vi "Test Find Chessboard Corners.vi"(8 "error in (no error)":errorcluster, 11 "Test Case In":refnum<class "02_FeatureDetection.lvclass">) -> (0 "error out":errorcluster, 3 "Test Case Out":refnum<class "02_FeatureDetection.lvclass">)   [LabVIEW 2020, in "test.lvlib" / "02_FeatureDetection.lvclass"]
uses:
  02_FeatureDetection.lvclass
  02_FeatureDetection.lvclass/02_FeatureDetection.ctl
  image/image.lvlib
  ar/ar.lvlib
  <vilib>/Astemes/LUnit/Test Case.lvclass
  common/Image Size (Integer).ctl
  common/common.lvlib
  ar/Chessboard Corner Info.ctl
  ar/Find Chessboard Corners (Greyscale).vi
  image/Draw Circle (Greyscale).vi
  image/Draw Image to Picture (Greyscale).vi
  common/Image Point (Float).ctl
  image/Interpolation Mode.ctl
  image/New Image (Greyscale Preallocated).vi
  image/Resize (Greyscale).vi
  image/New Image (Greyscale Array).vi
  C:/Program Files (x86)/National Instruments/LabVIEW 2020/vi.lib/Astemes/LUnit/Test Case.lvclass
  C:/Program Files (x86)/National Instruments/LabVIEW 2020/vi.lib/Astemes/LUnit/LUnit Runnable.lvclass
  C:/serenial/lib/g-augmented-reality-toolkit/LabVIEW/test/FeatureDetection/02_FeatureDetection.lvclass
panel:
  out "Points":T1[](array[typedef])
  out "Points Refined":T1[](array[typedef])
  out "Picture":picture
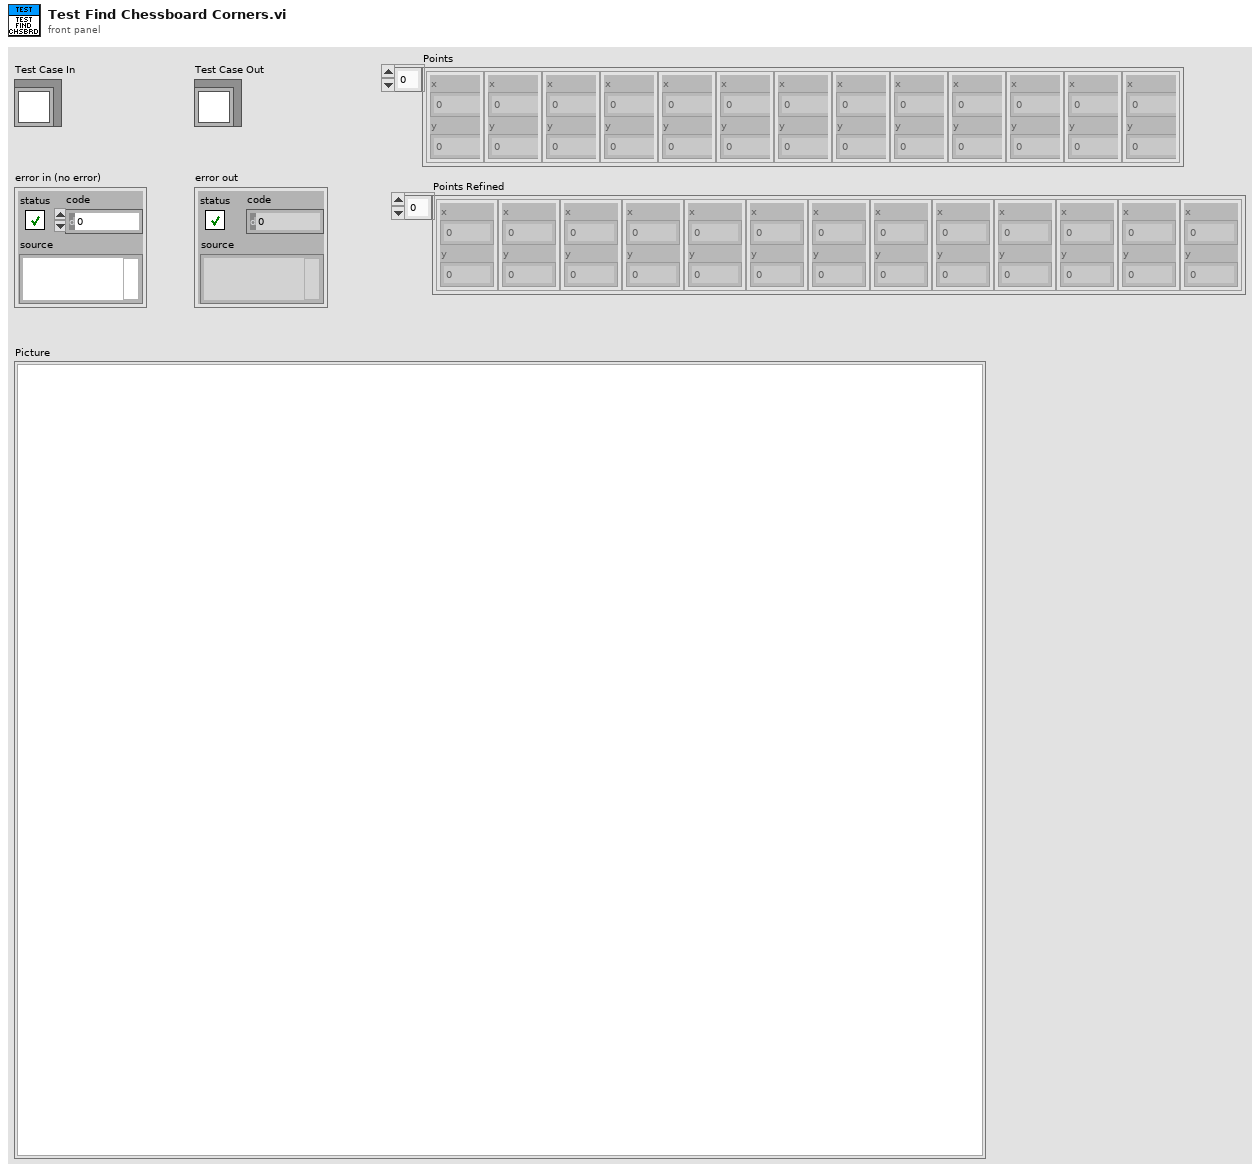
[diagram p1: front panel]
types:
  T1 = typedef "common.lvlib/Image Point (Float).ctl" = cluster{"x":dbl, "y":dbl}
  T2 = typedef "image.lvlib/Interpolation Mode.ctl" = enum8{"NEAREST", "LINEAR", "CUBIC", "AREA", "LANCZOS", "LINEAR_EXACT", "NEAREST_EXACT", "MAX"}
  T3 = typedef "ar.lvlib/Chessboard Corner Info.ctl" = cluster{"Points Per Row":u8, "Points Per Col":u8}
  T4 = typedef "common.lvlib/Image Size (Integer).ctl" = cluster{"Width":u16, "Height":u16}
  T5 = typedef "image.lvlib/Greyscale Image.ctl" = refnum<data-value>
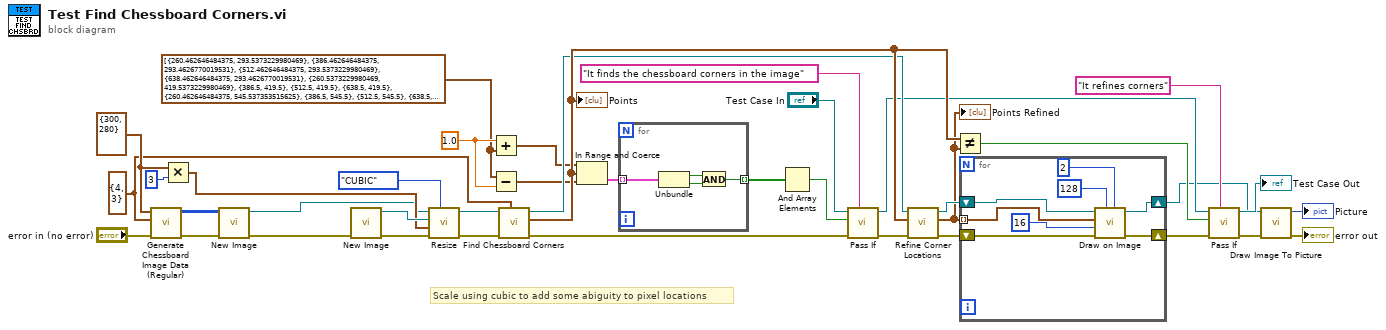
[diagram p0: block diagram]
diagram:
  w4 = T1[] [{"x"=260.462646484375, "y"=293.5373229980469}, {"x"=386.462646484375, "y"=293.4626770019531}, {"x"=512.462646484375, "y"=293.5373229980469}, {"x"=638.462646484375, "y"=293.4626770019531}, {"x"=260.5373229980469, "y"=419.5373229980469}, {"x"=386.5, "y"=419.5}, {"x"=512.5, "y"=419.5}, {"x"=638.5, "y"=419.5}, {"x"=260.462646484375, "y"=545.537353515625}, {"x"=386.5, "y"=545.5}, {"x"=512.5, "y"=545.5}, {"x"=638.5, "y"=545.5}] ("Points")
  w3 = T3 {"Points Per Row"=4, "Points Per Col"=3} ("Chessboard Corners Info")
  w28 = T4 {"Width"=300, "Height"=280} ("Target Size")
  w10 = 1.0
  # "Scale using cubic to add some abiguity to pixel locations"
  n1 = call "Generate Chessboard Image Data (Regular).vi"("error in (no error)"="error in (no error)", "Chessboard Corners Info"=w3, "Target Size"=w28) -> ("error out"=w34:errorcluster, "Chessboard Image Data"=w2:u8[][])  [unwired: 7 in]
  n2 = Multiply(x=w28, y=3) -> (x*y=w27:cluster{"Width":i32, "Height":i32})
  n3 = call-poly "New Image.vi"("error in (no error)"=w34, "U8 Greyscale Data"=w2) -> ("error out"=w32:errorcluster, "Greyscale Image"=w1:T5)  [unwired: 8 in]
  n4 = call-poly "New Image.vi"("error in (no error)"=w32) -> ("error out"=w30:errorcluster, "Greyscale Image"=w31:T5)  [unwired: 9 in]
  n5 = call-poly "Resize.vi"("Interpolation Mode (Default: CUBIC)"=Interpolation_Mode."CUBIC" ("OpenCV Interpolation Flag"), "error in (no error)"=w30, "New Image Size"=w27, "Greyscale Destination Image in"=w31, "Greyscale Source Image in"=w1) -> ("error out"=w29:errorcluster, "Greyscale Destination Image"=w25:T5)  [unwired: 5 in]
  n6 = Add(x=w10, y=w4) -> (x+y=w22:T1[])
  n7 = Subtract(x=w4, y=w10) -> (x-y=w23:T1[])
  n8 = call-poly "Find Chessboard Corners.vi"("Chessboard Corners Info"=w3, "error in (no error)"=w29, "Greyscale Image in"=w25) -> ("error out"=w39:errorcluster, "Points"=w38:T1[], "Greyscale Image"=w35:T5)  [unwired: 6 in]
  "Points" <- w38
  n9 = In Range and Coerce(upper limit=w22, x=w38, lower limit=w23) -> (In Range?=w21:cluster{"x":bool, "y":bool}[])  [unwired: 1 out]
  n10 = for {
    tunnel: w21 -> [w43] mode=indexing
    tunnel: [w40] -> w20 mode=indexing
    n11 = Unbundle(w43) -> ("x"=w42:bool, "y"=w41:bool)
    n12 = And(x=w42, y=w41) -> (x .and. y?=w40:bool)
  }
  n13 = And Array Elements(Boolean array=w20) -> (logical AND=w19:bool)
  n14 = call <vilib>:"Pass If.vi"("Description"="It finds the chessboard corners in the image", "error in (no error)"=w39, "Pass?"=w19, "LUnit Test Case In"="Test Case In") -> ("error out"=w16:errorcluster, "LUnit Test Case Out"=w14:refnum<class "02_FeatureDetection.lvclass">)  [unwired: 6 in]
  n15 = call "Refine Corner Locations.vi"("error in (no error)"=w16, "Points in"=w38, "Greyscale Image in"=w35) -> ("error out"=w8:errorcluster, "Points out"=w5:T1[], "Greyscale Image"=w9:T5)  [unwired: 6 in]
  "Points Refined" <- w5
  n16 = Not Equal?(x=w38, y=w5) -> (x != y?=w12:bool)
  n17 = for {
    shift-right: [w48] -> w6
    shift-left: w9 -> [w51]
    shift-right: [w49] -> w7
    shift-left: w8 -> [w50]
    tunnel: w5 -> [w47] mode=indexing
    n18 = call-poly "Draw on Image.vi"("Thickness (Default: 1)"=2, "Colour"=u8 128, "error in (no error)"=w50, "Radius"=u16 16, "Centre"=w47, "Greyscale Image in"=w51) -> ("error out"=w49:errorcluster, "Greyscale Image"=w48:T5)  [unwired: 4 in]
  }
  n19 = call <vilib>:"Pass If.vi"("Description"="It refines corners", "error in (no error)"=w7, "Pass?"=w12, "LUnit Test Case In"=w14) -> ("error out"=w15:errorcluster, "LUnit Test Case Out"=→"Test Case Out":refnum<class "02_FeatureDetection.lvclass">)  [unwired: 6 in]
  n20 = call-poly "Draw Image To Picture.vi"("error in (no error)"=w15, "Greyscale Image Source in"=w6) -> ("error out"=→"error out":errorcluster, "Picture"=→"Picture":picture)  [unwired: 8 in]
